vi "h.ACQ.GetStreamingPeaks.vi"(8 "error in":errorcluster, 10 "Timeout":i32=10000, 11 "Connection ID In":refnum<k5>) -> (0 "error out":errorcluster, 2 "Peaks Data":T2 {"Peaks Wvls, nm"."Peak Wvls, nm" format="%#_8g"}, 3 "Connection ID Out":refnum<k5>)   [LabVIEW 2016, in "h.Library.lvlib"]
doc: "This vi retrieves data from a streaming data socket.\n\n<b>Connection ID In</b> - is a network connection refnum that uniquely identifies the TCP connection\n<b>Timeout</b> - specifies the maximum amount of time, in milliseconds, for the function to complete\n<b>error in</b> - describes error conditions that occur before this node runs. This input provides standard error functionality\n<b>Connection ID Out</b> - returns the same value as connection ID\n<b>Peaks Data</b> - peaks wvl data\n<b>error out</b> - contains error information. This output provides standard error out functionality."
uses:
  h.Library.lvlib
  CTL/h.ACQ.PeaksData.ctl
  CTL/h.ACQ.PeaksWvl.ctl
  COMM/CTL/h.COMM.Command Status Enum.ctl
  COMM/CTL/h.COMM.Socket Type.ctl
panel:
  out "Status":T1
  # "Hyperion Get Streaming Peaks"
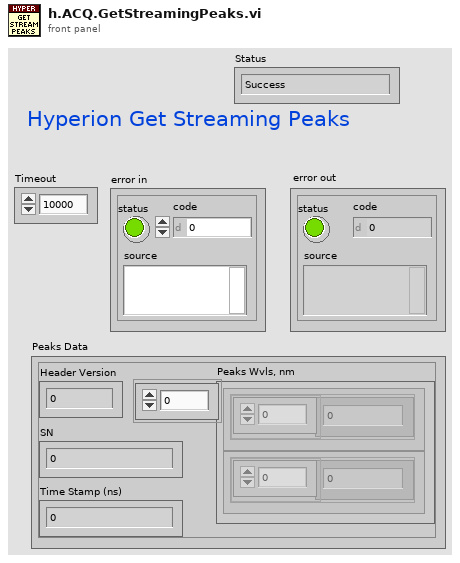
[diagram p1: front panel]
types:
  T1 = typedef "h.Library.lvlib/h.COMM.Command Status Enum.ctl" = enum8{"Success", "Failed", "Error", "AccessDenied", "InvalidCommand", "InvalidNumberArguments", "InvalidArgument", ""}
  T2 = typedef "h.Library.lvlib/h.ACQ.PeaksData.ctl" = cluster{"SN":u64, "Time Stamp (ns)":u64, "Header Version":u16, "Peaks Wvls, nm":T3[]}
  T3 = typedef "h.Library.lvlib/h.ACQ.PeaksWvl.ctl" = cluster{"Peak Wvls, nm":dbl[]}
  T4 = typedef "h.Library.lvlib/h.COMM.Socket Type.ctl" = u16
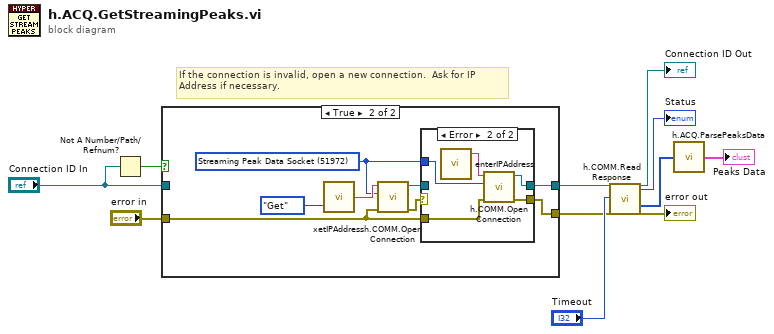
[diagram p0: block diagram]
diagram:
  # "If the connection is invalid, open a new connection.  Ask for IP\nAddress if necessary."
  n1 = Not A Number/Path/Refnum?(number/path/refnum="Connection ID In") -> (NaN/Path/Refnum?=w5:bool)
  n2 = case shown="True" w5 {
    tunnel: "Connection ID In" -> [w13 _]
    tunnel: [w13 w17] -> w3
    tunnel: "error in" -> [w12 w15]
    tunnel: [w12 w14] -> w1
    frame False {
    }
    frame True {
      w16 = T4 51972 items=["Command Socket"=51971, "Streaming Peak Data Socket"=51972, "Streaming Spectral Data Socket"=51973, "Streaming Sensor Data Socket"=51974] ("Port")
      n3 = call "xetIPAddress.vi"("Get/Set"=enum16{"Get", "Set"}."Get") -> ("IP Address Out"=w20:string)  [unwired: 1 in]
      n4 = call "h.COMM.Open Connection.vi"("error in"=w15, "Port"=w16, "Address"=w20) -> ("error out"=w19:errorcluster, "Connection ID"=w18:refnum<k5>)  [unwired: 7 in]
      n5 = case shown="Error" w19 {
        selector: w19 -> [w22 _]
        tunnel: w18 -> [w23 _]
        tunnel: [w23 w27] -> w17
        tunnel: w16 -> [_ w26]
        tunnel: [w22 w24] -> w14
        tunnel: w15 -> [_ w25]
        frame No Error {
        }
        frame Error {
          n6 = call "enterIPAddress.vi"() -> ("IP Address Out"=w28:string)  [unwired: 2 in, 1 out]
          n7 = call "h.COMM.Open Connection.vi"("error in"=w25, "Port"=w26, "Address"=w28) -> ("error out"=w24:errorcluster, "Connection ID"=w27:refnum<k5>)  [unwired: 7 in]
        }
      }
    }
  }
  n8 = call "h.COMM.Read Response.vi"("Connection ID"=w3, "Timeout"="Timeout", "error in"=w1) -> ("Connection ID"=→"Connection ID Out":refnum<k5>, "Status"=→"Status":T1, "Content"=w8:u8[], "error out"=→"error out":errorcluster)  [unwired: 17 in, 4 out]
  n9 = call "h.ACQ.ParsePeaksData.vi"("Data from #GetPeaks"=w8) -> ("Peaks Data"=→"Peaks Data":T2)
